vi "Cleanup.vi"(8 "error in (no error)":errorcluster, 11 "ButtonControlEditorPanel in":refnum<class "ButtonControlEditorPanel.lvclass">) -> (0 "error out":errorcluster)   [LabVIEW 2020]
uses:
  ButtonControlEditorPanel.lvclass
  ElementEditorPanel/ElementEditorPanel.lvclass
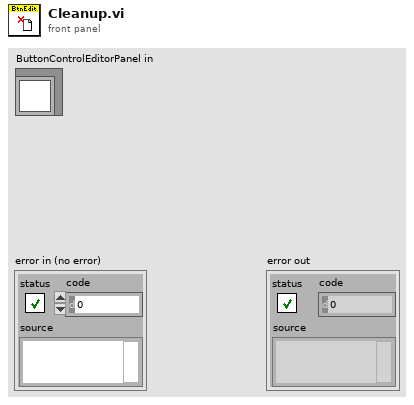
[diagram p1: front panel]
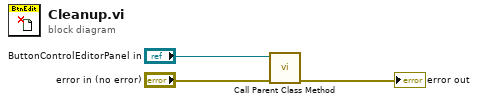
[diagram p0: block diagram]
diagram:
  n1 = call-parent "Call Parent Class Method"("error in (no error)"="error in (no error)", "ElementEditorPanel in"="ButtonControlEditorPanel in") -> ("error out"=→"error out":errorcluster)  [unwired: 9 in]
